vi "Recieve DAQ Data From Notifier.vi"(1 "Notifier Name":string) -> (0 "Experimental Data":dbl[][](array[numeric]))   [LabVIEW 2013]
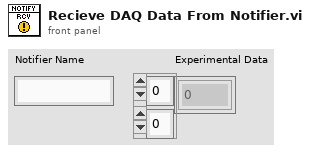
[diagram p1: front panel]
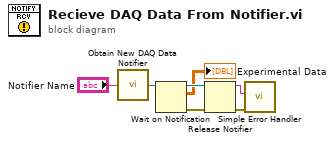
[diagram p0: block diagram]
diagram:
  n1 = call "Obtain New DAQ Data Notifier.vi"("Notifier Name"="Notifier Name") -> ("DAQ Data Notifier"=w6:refnum<notifier>)
  n2 = Wait on Notification(notifier=w6) -> (notifier out=w3:refnum<notifier>, notification=→"Experimental Data":dbl[][], error out=w2:errorcluster)  [unwired: 3 in, 1 out]
  n3 = Release Notifier(notifier=w3, error in (no error)=w2) -> (notifier name=w4:string, error out=w5:errorcluster)  [unwired: 1 in, 1 out]
  n4 = call <vilib>:"Simple Error Handler.vi"("error source (\" \")"=w4, "error in (no error)"=w5) -> ()  [unwired: 3 in, 5 out]
